vi "PXI_Host_LargeFXP_Read_NewMethod_Benchmark.vi"() -> ()   [LabVIEW 2018]
uses:
  <vilib>/Platform/TimedLoop/XDataNode/timing_clust.ctl
  <vilib>/Platform/TimedLoop/XDataNode/nitl_modes.ctl
  <vilib>/Platform/TimedLoop/XDataNode/wakeup.ctl
  cRIO RT/FPGA Bitfile Register Operations/Scalar IO Operations/TypeDefs/FXP Configuration.ctl
  <vilib>/fxp/LVFixedPointRepBitsTypeDef.ctl
  <vilib>/fxp/LVFixedPointRepRangeTypeDef.ctl
  cRIO RT/FPGA Bitfile Register Operations/Scalar IO Operations/SubVIs/FXP Raw to DBL.vi
  cRIO RT/FPGA Bitfile Register Operations/Scalar IO Operations/Read Methods/Read Data Register/Instances/Read U16.vi
  cRIO RT/FPGA Bitfile Register Operations/Scalar IO Operations/Read Methods/Read Data Register/Instances/Read U32.vi
  cRIO RT/FPGA Bitfile Register Operations/Scalar IO Operations/Read Methods/Read Data Register/Instances/Read U64.vi
  cRIO RT/FPGA Bitfile Register Operations/Scalar IO Operations/Read Methods/Read Data Register/Instances/Read U8.vi
  cRIO RT/FPGA Bitfile Register Operations/Scalar IO Operations/Utilities/Find Register Offset.vi
  cRIO RT/FPGA Bitfile Register Operations/Scalar IO Operations/SubVIs/Check Register Data Store.vi
  cRIO RT/FPGA Bitfile Register Operations/Scalar IO Operations/Error Handling/Error 6001.vi
  cRIO RT/FPGA Bitfile Register Operations/Scalar IO Operations/Error Handling/Error 6000.vi
  cRIO RT/FPGA Bitfile Register Operations/Scalar IO Operations/Error Handling/Error 6002.vi
  cRIO RT/FPGA Bitfile Register Operations/Scalar IO Operations/Error Handling/Error 6003.vi
  <vilib>/FPGAPlugInAG/Dynamic/niLvFpga_Close_Dynamic.vi
  <vilib>/platform/TimedLoop/XDataNode/XDataNode.xnode
  <vilib>/rvi/interface/nirviCloseFPGA/nirviCloseFPGA.xnode
  cRIO RT/FPGA Bitfile Register Operations/Scalar IO Operations/Read Methods/Read Data Register/Instances/Read FXP.vi
  cRIO RT/FPGA Bitfile Register Operations/Scalar IO Operations/FPGA Register IO.lvlib
  <vilib>/Platform/TimedLoop/XDataNode/XDNodeRunTimeDep.lvlib
panel:
  out "Waveform Graph":dbl[](graph)
  out "Standard Dev":dbl
  out "Arithmetic Mean":dbl
  out "Maximum":dbl
  out "DBL Value":dbl
  out "error out":errorcluster
  # "Recorded time"
  # "3.37551E-5"
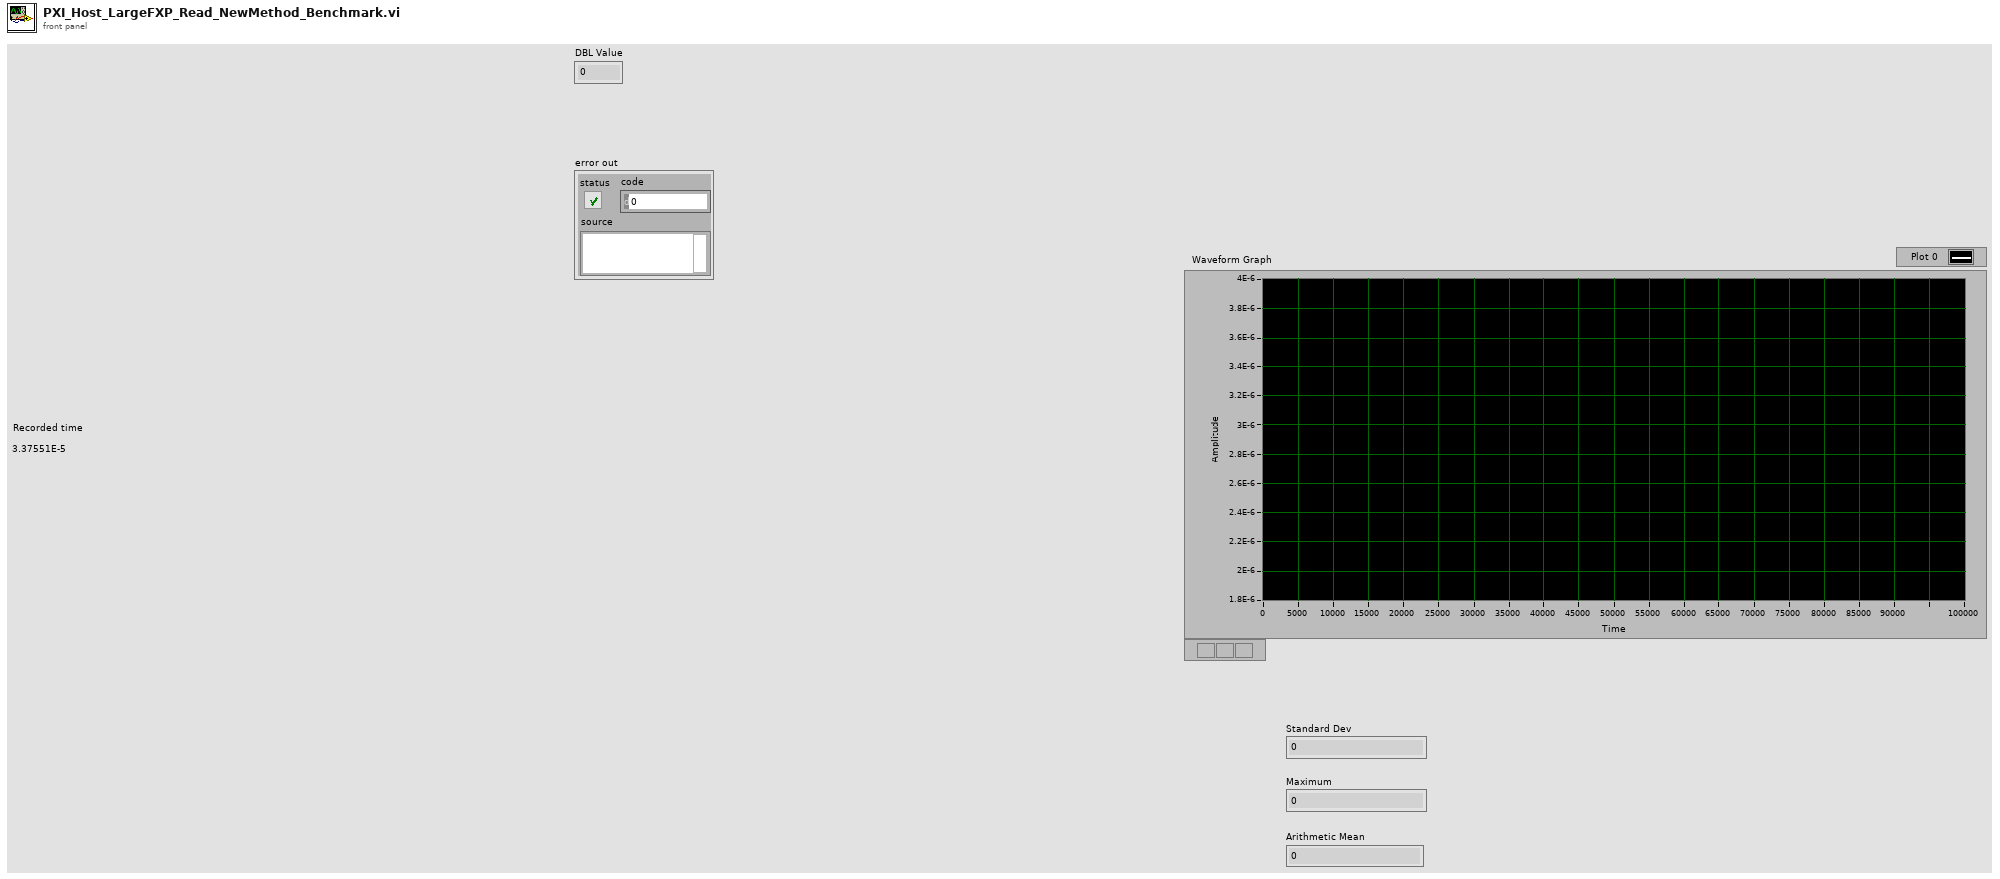
[diagram p1: front panel]
types:
  T1 = typedef "XDNodeRunTimeDep.lvlib/timing_clust.ctl" = cluster{"Expected End [f-1]":u64, "Actual End [f-1]":u64, "Finished Late? [f-1]":bool, "Expected End [i-1]":u64, "Actual End [i-1]":u64, "Finished Late? [i-1]":bool, "Expected Start [i]":u64, "Actual Start [i]":u64, "Expected Start [f]":u64, "Actual Start [f]":u64, "Source Name":string, "Structure Name":string, "Period":i64, "Deadline":i64, "Offset":i64, "Start":i64, "Priority":i32, "Timeout":i32, "Mode":T2, "Wakeup Reason":T3, "Error":errorcluster, "Source Type":string, "Secondary Source Type":string, "Global End Time":u64, "Global Start Time":u64, "Frame Duration":u64, "Iteration Duration":u64, "Assigned CPU":i32, "I/O Scan Engine Mode":u32}
  T2 = typedef "XDNodeRunTimeDep.lvlib/nitl_modes.ctl" = enum32{"No Change", "Process missed periods, maintain original phase", "Discard missed periods, maintain original phase", "Process missed periods, ignore original phase", "Discard missed periods, ignore original phase"}
  T3 = typedef "XDNodeRunTimeDep.lvlib/wakeup.ctl" = enum32{"Normal", "Aborted", "Asynchronous wakeup", "Timing source error", "Timed loop error", "Timeout"}
  T4 = typedef "FPGA Register IO.lvlib/FXP Configuration.ctl" = cluster{"FXP Representation":T5, "FXP Range":T6}
  T5 = typedef "LVFixedPointRepBitsTypeDef.ctl" = cluster{"Signed":bool, "Word Length":u32, "Integer Word Length":i32}
  T6 = typedef "LVFixedPointRepRangeTypeDef.ctl" = cluster{"Range Min":dbl, "Range Max":dbl, "Delta":dbl}
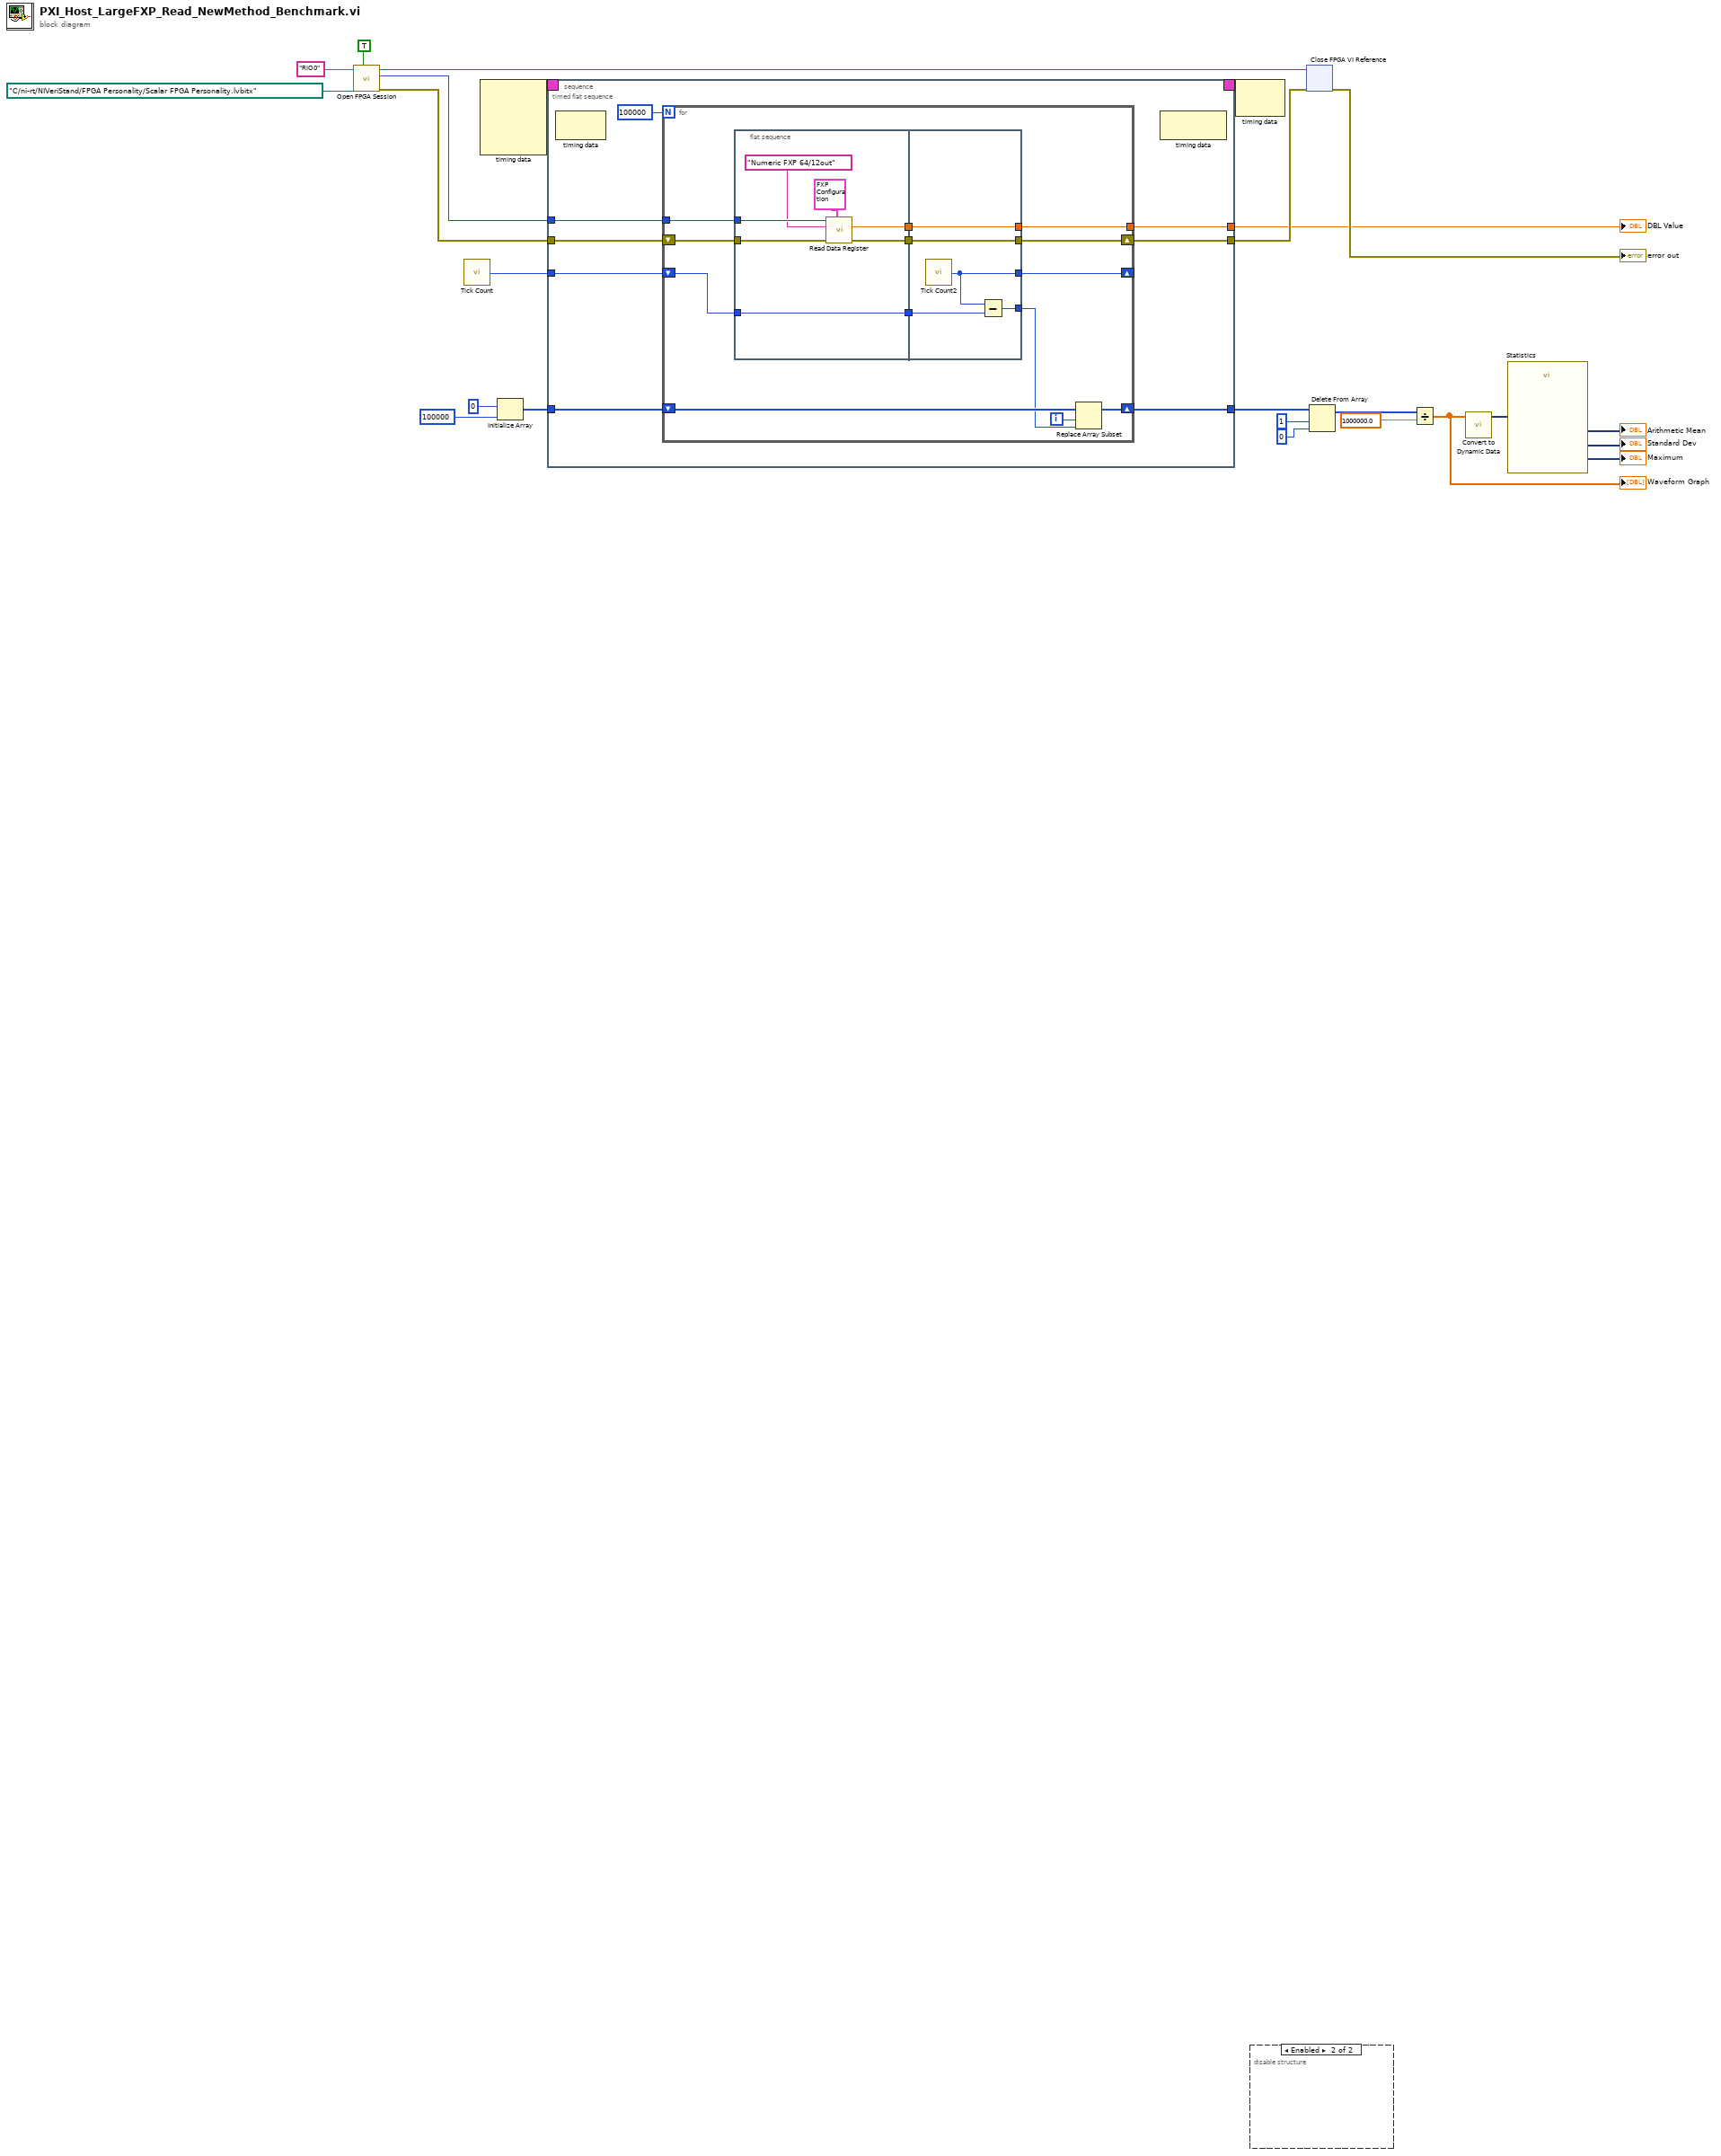
[diagram p0: block diagram]
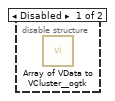
[diagram p2: hidden frame]
diagram:
  n1 = call "Open FPGA Session.vi"("run when loaded (T)"=TRUE, "bitfile path"=path "C:/ni-rt/NIVeriStand/FPGA Personality/Scalar FPGA Personality.lvbitx", "device address"="RIO0") -> ("error out"=w21:errorcluster, "session out"=w25:u32, "bitfile reference out"=w20:refnum<k20>)  [unwired: 6 in]
  n2 = call "Tick Count"() -> ("Tick Count(uSec)"=w14:u32)
  n3 = node-c288() -> (w16:T1)  [unwired: 4 in]
  n4 = Initialize Array(u32 0 ("Tick Count(uSec)"), 100000) -> (w11:u32[])
  n5 = timed-sequence {
    timing: w16 -> [_]
    timing-out: [_] -> w15
    tunnel: w25 -> [w32]
    tunnel: w21 -> [w31]
    tunnel: [w30] -> w19
    tunnel: [w29] -> w17
    tunnel: w14 -> [w28]
    tunnel: w11 -> [w27]
    tunnel: [w26] -> w1
    n6 = timed-flat-sequence {
      tunnel: w32 -> [w40]
      tunnel: w31 -> [w39]
      tunnel: [w38] -> w30
      tunnel: [w37] -> w29
      tunnel: w28 -> [w35]
      tunnel: w27 -> [w34]
      tunnel: [w33] -> w26
      n7 = node-c288() -> ()  [unwired: 1 in, 1 out]
      n8 = for {
        N: 100000 -> [_]
        tunnel: w40 -> [w51]
        tunnel: [w48] -> w37
        shift-right: [w49] -> w38
        shift-left: w39 -> [w50]
        shift-right: [w45] -> _
        shift-left: w35 -> [w47]
        shift-right: [w41] -> w33
        shift-left: w34 -> [w44]
        i -> [w43]
        n9 = flat-sequence {
          tunnel: [w58] -> w53
          tunnel: [w57] -> w52
          tunnel: w51 -> [w60]
          tunnel: w50 -> [w59]
          tunnel: w47 -> [w54]
          tunnel: [w54] -> w46
          tunnel: [w65] -> w42
          tunnel: w53 -> [w64]
          tunnel: [w64] -> w49
          tunnel: w52 -> [w63]
          tunnel: [w63] -> w48
          tunnel: w46 -> [w62]
          tunnel: [w61] -> w45
          frame #0 {
            n10 = call-poly "Read Data Register.vi"("FXP Configuration"=T4 {"FXP Representation"={"Signed"=TRUE, "Word Length"=64, "Integer Word Length"=12}, "FXP Range"={"Range Min"=-2048.0, "Range Max"=2048.0, "Delta"=2.22045e-16}}, "error in"=w59, "register name"="Numeric FXP 64/12out", "session in"=w60) -> ("error out"=w58:errorcluster, "DBL Value"=w57:dbl)  [unwired: 5 in, 1 out]
          }
          frame #1 {
            n11 = call "Tick Count2"() -> ("Tick Count(uSec)"=w61:u32)
            n12 = Subtract(x=w61, y=w62) -> (x-y=w65:u32)
          }
        }
        n13 = Replace Array Subset(array=w44, new element=w42, index=w43) -> (w41:u32[])
      }
      n14 = node-c288() -> ()  [unwired: 1 in, 1 out]
    }
  }
  "DBL Value" <- w17
  n15 = node-c288(w15) -> ()  [unwired: 1 out]
  n16 = disable-structure shown="Enabled" {
    frame Disabled {
      n17 = call <userlib>:"Array of VData to VCluster__ogtk.vi"() -> ()  [unwired: 10 in, 2 out]
    }
    frame Enabled {
    }
  }
  n18 = xnode "Close FPGA VI Reference"("FPGA VI Reference In"=w20, "error in"=w19) -> ("error out"=→"error out":errorcluster)
  n19 = Delete From Array(array=w1, length=1, index=0) -> (array with subset deleted=w2:u32[])  [unwired: 1 out]
  n20 = Divide(x=w2, y=1000000.0) -> (x/y=w3:dbl[])
  "Waveform Graph" <- w3
  n21 = call "Convert to Dynamic Data"("Array"=w3) -> ("Dynamic Data Type"=w10:dynamicdata)  [unwired: 3 in]
  n22 = call "Statistics"("Signals"=w10) -> ("Standard Dev"=→"Standard Dev":dynamicdata, "Arithmetic Mean"=→"Arithmetic Mean":dynamicdata, "Maximum"=→"Maximum":dynamicdata)  [unwired: 23 in, 1 out]
